vi "Statistical measure - basics - 1.vi"(5 "Data measured":dbl[](array[numeric]), 9 "Data reference":dbl[](array[numeric])) -> (3 "x != y?":bool, 8 "Statistcs":T1 {"mean meas" format="%.10f"; "min meas" format="%.10f"; "max meas" format="%.10f"; "mean dev" format="%.10f"; "min dev" format="%.10f"; "max dev" format="%.10f"; "mean ref" format="%.10f"; "min ref" format="%.10f"; "max ref" format="%.10f"})   [LabVIEW 2020]
panel:
  # "Statistical Measure - Basics - 1"
  # "array size"
  # "Deviaton"
  # "Measured"
  # "Reference"
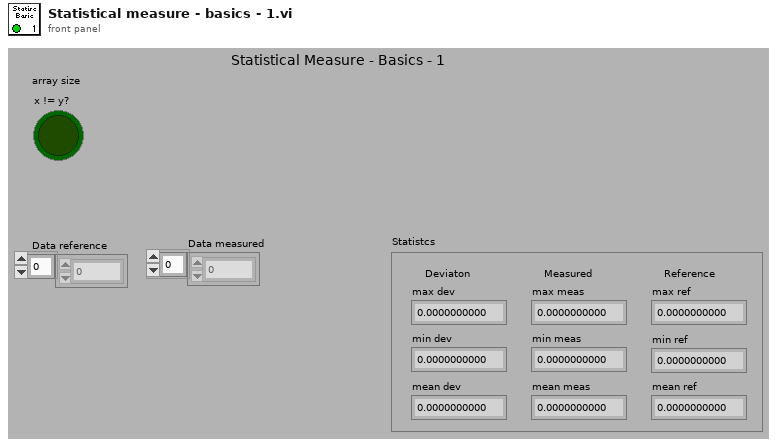
[diagram p1: front panel]
types:
  T1 = cluster{"max ref":dbl, "min ref":dbl, "mean ref":dbl, "max dev":dbl, "min dev":dbl, "mean dev":dbl, "max meas":dbl, "min meas":dbl, "mean meas":dbl}
  T2 = cluster{dbl, dbl, dbl, dbl, dbl, dbl, dbl, dbl, dbl}
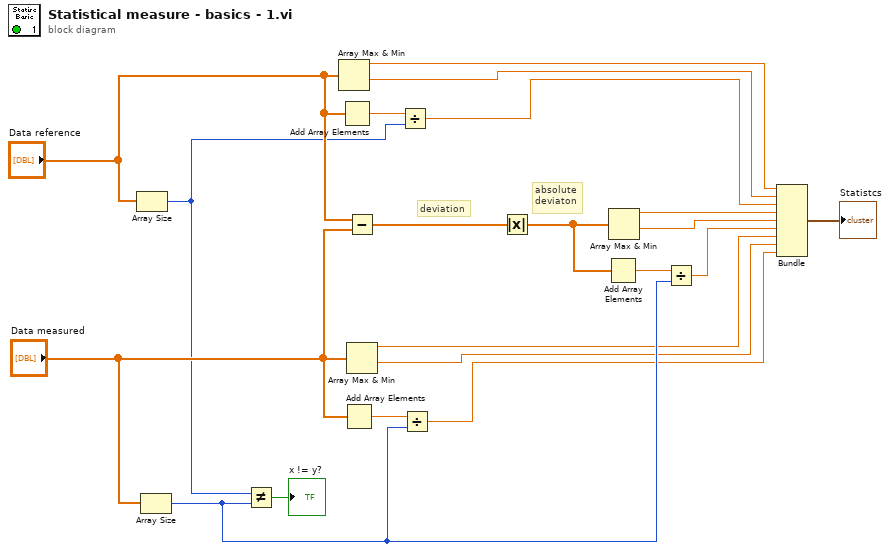
[diagram p0: block diagram]
diagram:
  # "deviation"
  # "absolute\ndeviaton"
  n1 = Array Size(array="Data reference") -> (size(s)=w11:i32)
  n2 = Array Size(array="Data measured") -> (size(s)=w14:i32)
  n3 = Not Equal?(x=w11, y=w14) -> (x != y?=→"x != y?":bool)
  n4 = Array Max & Min(array="Data reference") -> (max value=w9:dbl, min value=w8:dbl)  [unwired: 2 out]
  n5 = Add Array Elements(numeric array="Data reference") -> (sum=w13:dbl)
  n6 = Add Array Elements(numeric array="Data measured") -> (sum=w16:dbl)
  n7 = Subtract(x="Data reference", y="Data measured") -> (x-y=w20:dbl[])
  n8 = Array Max & Min(array="Data measured") -> (max value=w3:dbl, min value=w2:dbl)  [unwired: 2 out]
  n9 = Divide(x=w13, y=w11) -> (x/y=w7:dbl)
  n10 = Divide(x=w16, y=w14) -> (x/y=w1:dbl)
  n11 = Absolute Value(x=w20) -> (abs(x)=w18:dbl[])
  n12 = Add Array Elements(numeric array=w18) -> (sum=w17:dbl)
  n13 = Array Max & Min(array=w18) -> (max value=w6:dbl, min value=w5:dbl)  [unwired: 2 out]
  n14 = Divide(x=w17, y=w14) -> (x/y=w4:dbl)
  n15 = Bundle(w9, w8, w7, w6, w5, w4, w3, w2, w1) -> (→"Statistcs":T2)  [unwired: 1 in]
